vi "Tree_Cluster Element to Tag.vi"(10 "Index":i32, 11 "Cluster Element Data":T1) -> (2 "Tree Tag Value":string, 3 "Cluster Element Data Out":T1)   [LabVIEW 2023]
doc: "Builds a \".\" delimited string from the Nest Chain and Element Label. If the nest chain is empty, the element label is output. Thus, if the element label already represents the nest chain, or is the top level item, this function does what it's supposed to do.\n\nCreate Tree Tag value if it doesn't already appear in cluster."
uses:
  cluster/Cluster Element Description.ctl
  <vilib>/Utility/error.llb/Trim Whitespace One-Sided.vi
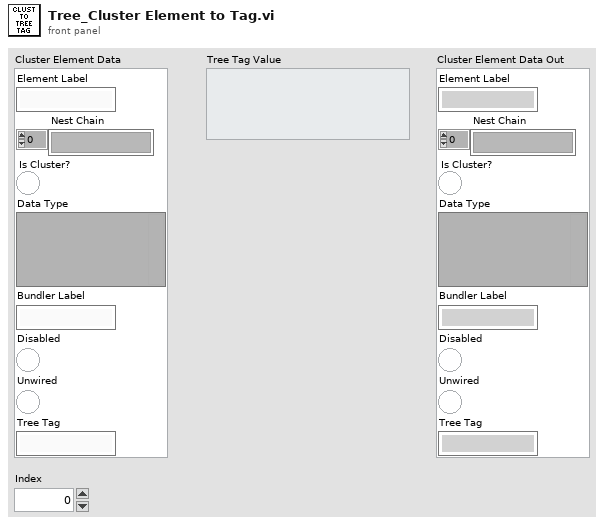
[diagram p1: front panel]
types:
  T1 = typedef "Cluster Element Description.ctl" = cluster{"Element Label":string, "Nest Chain":string[], "Is Cluster?":bool, "Data Type":variant, "Bundler Label":string, "Disabled":bool, "Unwired":bool, "Tree Tag":string}
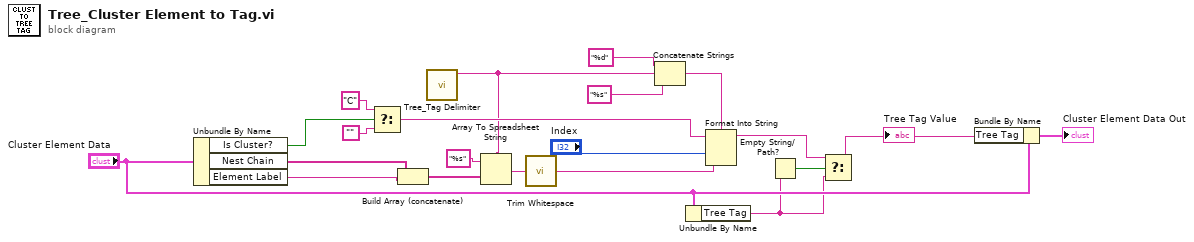
[diagram p0: block diagram]
diagram:
  n1 = Unbundle By Name("Cluster Element Data") -> ("Is Cluster?"=w20:bool, "Nest Chain"=w10:string[], "Element Label"=w9:string)
  n2 = Select(t="C", s=w20, f="") -> (s? t:f=w18:string)
  n3 = Build Array (concatenate)(w10, w9) -> (w11:string[])
  n4 = call "Tree_Tag Delimiter.vi"() -> ("Tree Tag delimiter"=w7:string)  [unwired: 11 in]
  n5 = Array To Spreadsheet String(delimiter (Tab)=w7, array=w11, 3:"%s" ("format string")) -> (spreadsheet string=w12:string)
  n6 = call <vilib>:"Trim Whitespace.vi"("string"=w12) -> ("trimmed string"=w8:string)  [unwired: 1 in]
  n7 = Concatenate Strings("%d", w7, "%s") -> (w14:string)
  n8 = Unbundle By Name("Cluster Element Data") -> ("Tree Tag"=w4:string)
  n9 = Format Into String(format string=w14, initial string=w18, "Index", w8) -> (resulting string=w2:string)  [unwired: 1 in, 1 out]
  n10 = Empty String/Path?(string/path=w4) -> (empty?=w3:bool)
  n11 = Select(t=w2, s=w3, f=w4) -> (s? t:f=w1:string)
  "Tree Tag Value" <- w1
  n12 = Bundle By Name(cluster="Cluster Element Data", "Tree Tag"=w1) -> (→"Cluster Element Data Out":T1)
